vi "AC_CmdStr_2F2.vi"(1 "AC命令输入":T1={"自动请求状态"=FALSE, "空调按键引起弹窗显示"=FALSE, "最大制冷请求状态"=FALSE, "除霜请求状态"=FALSE, "内外循环进气"=0, "空气质量传感器请求"=FALSE, "吹风档位"=0, "负离子发生器状态"=0, "吹风模式"=0, "空调开启状态"=FALSE, "左侧设定温度"=18.0, "空调开关按键音"=FALSE, "AC远程控制模式与否"=FALSE, "空调按键触摸状态"=0, "空调按键状态"=0} {"空调按键状态" items=["No Press", "Blowup", "BlowDown", "AC Req", "MaxAcReq", "AUTOreq", "DefrostReq", "RearDefReq", "AirDistributionModeReq", "CycleReq", "DualReq", "IONreq", "AqsReq", "LeftTempUp", "LeftTempDown", "RightTempUp", "RightTempDown", "OFF", "KeyBLW"]; "空调按键触摸状态" items=["No Touch", "KeyLeftTemp", "KeyRightTemp", "KeyAUTO", "KeyAC", "KeyBLW+", "KeyBLW-", "KeyMODE", "KeyDEF", "KeyRearDEF", "KeyIntake", "KeyBLW", "Reserved"]; "左侧设定温度" min=17.5 max=31.5 step=0.5 scale=17.5..31.5 scale format="%#_6f"; "吹风模式" items=["Face", "Bilevel", "Foot", "FootScreen", "Screen", "预留", "无效"]; "负离子发生器状态" items=["关闭", "开启", "预留", "错误"]; "吹风档位" items=["关闭", "等级1", "等级2", "等级3", "等级4", "等级5", "等级6", "等级7", "等级8", "无效"]; "内外循环进气" items=["Fresh", "循环", "保持", "无效"]}) -> (0 "CmdStr":string)   [LabVIEW 2013]
uses:
  AC_2F2.ctl
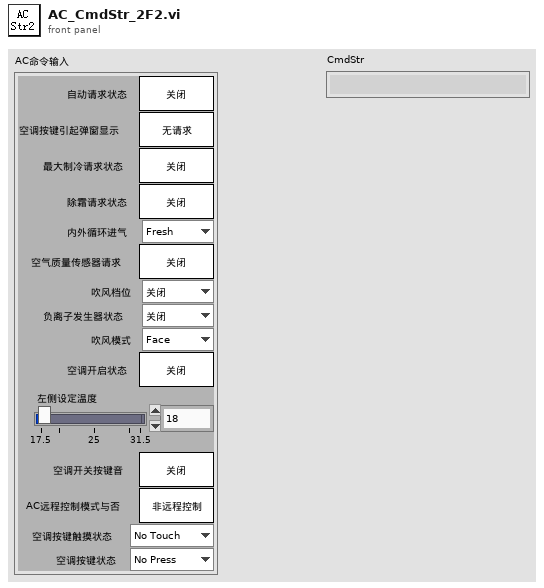
[diagram p1: front panel]
types:
  T1 = typedef "AC_2F2.ctl" = cluster{"自动请求状态":bool, "空调按键引起弹窗显示":bool, "最大制冷请求状态":bool, "除霜请求状态":bool, "内外循环进气":u16, "空气质量传感器请求":bool, "吹风档位":u16, "负离子发生器状态":u16, "吹风模式":u16, "空调开启状态":bool, "左侧设定温度":dbl, "空调开关按键音":bool, "AC远程控制模式与否":bool, "空调按键触摸状态":u16, "空调按键状态":u16}
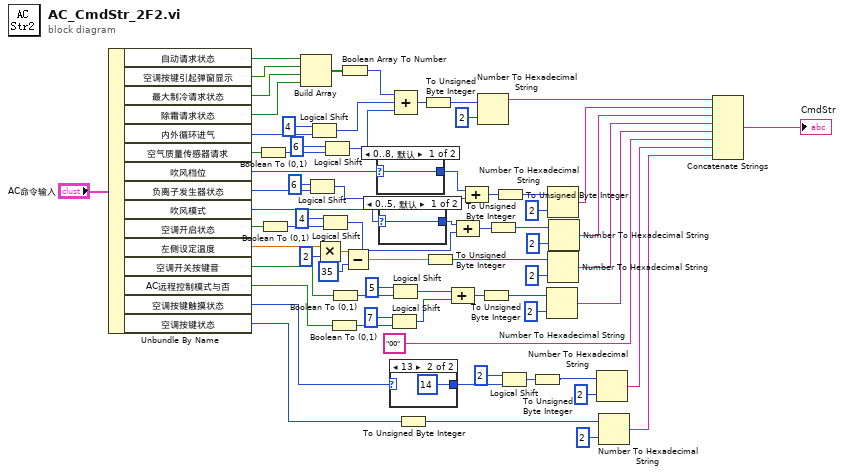
[diagram p0: block diagram]
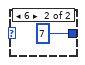
[diagram p3: hidden frame]
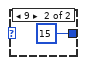
[diagram p4: hidden frame]
diagram:
  n1 = Unbundle By Name("AC命令输入") -> ("自动请求状态"=w69:bool, "空调按键引起弹窗显示"=w68:bool, "最大制冷请求状态"=w67:bool, "除霜请求状态"=w66:bool, "内外循环进气"=w65:u16, "空气质量传感器请求"=w61:bool, "吹风档位"=w55:u16, "负离子发生器状态"=w52:u16, "吹风模式"=w45:u16, "空调开启状态"=w48:bool, "左侧设定温度"=w42:dbl, "空调开关按键音"=w36:bool, "AC远程控制模式与否"=w33:bool, "空调按键触摸状态"=w29:u16, "空调按键状态"=w26:u16)
  n2 = Boolean To (0,1)(Boolean=w61) -> (0, 1=w59:i16)
  n3 = Boolean To (0,1)(Boolean=w48) -> (0, 1=w47:i16)
  n4 = Build Array(w69, w68, w67, w66) -> (w64:bool[])
  n5 = Logical Shift(y=u8 6, x=w52) -> (x << y=w51:u16)
  n6 = Logical Shift(y=u8 4, x=w65) -> (x << y=w62:u16)
  n7 = Multiply(x=w42, y=2) -> (x*y=w40:dbl)
  n8 = Logical Shift(y=u8 4, x=w47) -> (x << y=w44:i16)
  n9 = Logical Shift(y=u8 6, x=w59) -> (x << y=w57:i16)
  n10 = Boolean To (0,1)(Boolean=w33) -> (0, 1=w34:i16)
  n11 = Boolean To (0,1)(Boolean=w36) -> (0, 1=w38:i16)
  n12 = Boolean Array To Number(Boolean array=w64) -> (number=w63:u32)
  n13 = Subtract(x=w40, y=35) -> (x-y=w1:dbl)
  n14 = case shown="0..8, 默认" w55 {
    selector: w55 -> [w71 _]
    tunnel: [w71 u8 15] -> w54
    frame 0..8, Default {
    }
    frame 9 {
    }
  }
  n15 = case shown="0..5, 默认" w45 {
    selector: w45 -> [w73 _]
    tunnel: [w73 u8 7] -> w43
    frame 0..5, Default {
    }
    frame 6 {
    }
  }
  n16 = Logical Shift(y=u8 7, x=w34) -> (x << y=w31:i16)
  n17 = Logical Shift(y=u8 5, x=w38) -> (x << y=w32:i16)
  n18 = case shown="13" w29 {
    selector: w29 -> [w75 _]
    tunnel: [w75 u8 14] -> w28
    frame 0..12, Default {
    }
    frame 13 {
    }
  }
  n19 = Compound Arithmetic op=ADD(w63, w62, w57) -> (w56:u32)
  n20 = To Unsigned Byte Integer(number=w26) -> (unsigned 8bit integer=w4:u8)
  n21 = To Unsigned Byte Integer(number=w56) -> (unsigned 8bit integer=w22:u8)
  n22 = To Unsigned Byte Integer(number=w1) -> (unsigned 8bit integer=w13:u8)
  n23 = Compound Arithmetic op=ADD(w32, w31) -> (w30:i16)
  n24 = Compound Arithmetic op=ADD(w43, w44) -> (w46:u16)
  n25 = Compound Arithmetic op=ADD(w54, w51) -> (w50:u16)
  n26 = Number To Hexadecimal String(1:i16 2 ("宽度(-)"), 2:w22) -> (0:w23:string)
  n27 = To Unsigned Byte Integer(number=w30) -> (unsigned 8bit integer=w10:u8)
  n28 = To Unsigned Byte Integer(number=w46) -> (unsigned 8bit integer=w16:u8)
  n29 = To Unsigned Byte Integer(number=w50) -> (unsigned 8bit integer=w19:u8)
  n30 = Logical Shift(y=u8 2, x=w28) -> (x << y=w27:u16)
  n31 = To Unsigned Byte Integer(number=w27) -> (unsigned 8bit integer=w7:u8)
  n32 = Number To Hexadecimal String(1:i16 2 ("宽度(-)"), 2:w10) -> (0:w9:string)
  n33 = Number To Hexadecimal String(1:i16 2 ("宽度(-)"), 2:w19) -> (0:w18:string)
  n34 = Number To Hexadecimal String(1:i16 2 ("宽度(-)"), 2:w13) -> (0:w12:string)
  n35 = Number To Hexadecimal String(1:i16 2 ("宽度(-)"), 2:w16) -> (0:w15:string)
  n36 = Number To Hexadecimal String(1:i16 2 ("宽度(-)"), 2:w7) -> (0:w6:string)
  n37 = Number To Hexadecimal String(1:i16 2 ("宽度(-)"), 2:w4) -> (0:w3:string)
  n38 = Concatenate Strings(w23, w18, w15, w12, w9, "00", w6, w3) -> (→"CmdStr":string)
